vi "done Tx scenario.vi"(0 "all dds free":bool, 5 "done write files":bool, 9 "num of pulse sent to fpga":i32, 11 "pulse transmitted":u32[](array[numeric])) -> (4 "Checkbox out":bool)   [LabVIEW 2021]
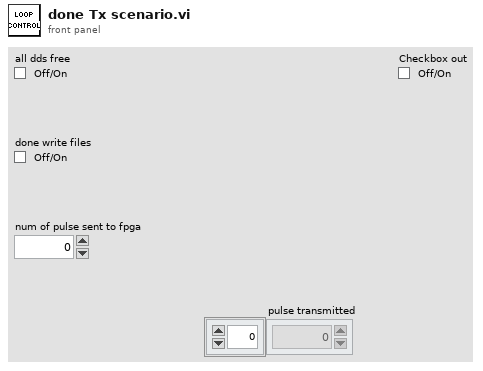
[diagram p1: front panel]
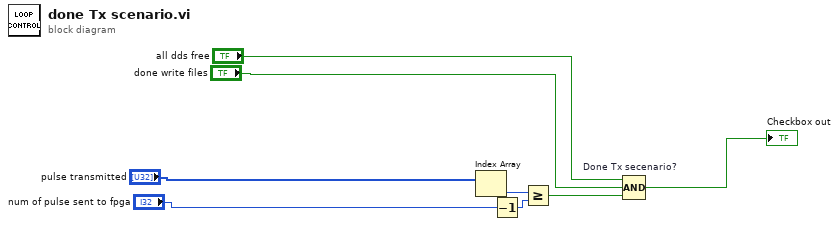
[diagram p0: block diagram]
diagram:
  n1 = Index Array(array="pulse transmitted") -> (element=w2:u32)  [unwired: 1 in]
  n2 = Decrement(x="num of pulse sent to fpga") -> (x-1=w3:i32)
  n3 = Greater Or Equal?(x=w2, y=w3) -> (x >= y?=w4:bool)
  n4 = Compound Arithmetic op=AND "Done Tx secenario?"("all dds free", "done write files", w4) -> (→"Checkbox out":bool)
